vi "main_particle-filter.vi"() -> ()   [LabVIEW 2019]
uses:
  <vilib>/Analysis/Matrix/Datatypes/RealMatrix.ctl
  Ctrl/cmd_common.ctl
  <vilib>/Analysis/baseanly.llb/Real A x B.vi
  <vilib>/Analysis/Matrix/Numeric/Add/Add (Elementwise) - RM,R.vi
  <vilib>/Analysis/Matrix/NI_Matrix.lvlib
  <vilib>/ptbypt/NI_PtbyPt.lvlib
  <vilib>/Analysis/NI_AALBase.lvlib
panel:
  in  "tab":enum32{"ini val", "observation val", "Param"}(tab)=enum."observation val"
  out "Q_sim":T1=[[0.04000000000000001]]
  out "R_sim":T1=[[1.0, 0.0], [0.0, 0.2741556778080377]]
  out "x_est":T1
  out "x_true":T1
  out "h_x_est":T1
  out "h_x_dr":T1 caption="x_true"
  out "h_x_true":T1 caption="x_true"
  out "x_dr":T1
  out "R":T1=[[4.0, 0.0], [0.0, 0.4873878716587337]]
  out "Q":T1=[[0.04000000000000001]]
  in  "rf_id":cluster{"x":dbl, "y":dbl}[](array[cluster])=[{"x"=10.0, "y"=0.0}, {"x"=10.0, "y"=10.0}, {"x"=0.0, "y"=15.0}, {"x"=-5.0, "y"=20.0}]
  in  "R est err-deg":dbl=40.0 format="%#_13g"
  in  "Q est range error":dbl=0.2 format="%#_13g"
  in  "R_sim error deg":dbl=30.0 format="%#_13g"
  in  "R est in-err-distance":dbl=2.0 format="%#_13g"
  in  "Q sim range err":dbl=0.2 format="%#_13g"
  in  "R_sim range":dbl=1.0 format="%#_13g"
  out "px old":T1
  out "px new":T1
  out "p_est":T1
  out "열의 개수":i32
  in  "DT":dbl=0.1
  in  "MAX_RANGE":dbl=20.0
  in  "SIM_TIME":dbl=50.0
  in  "NTh":u32=50
  in  "NP":u32=100
  out "time":dbl
  in  "정지":bool
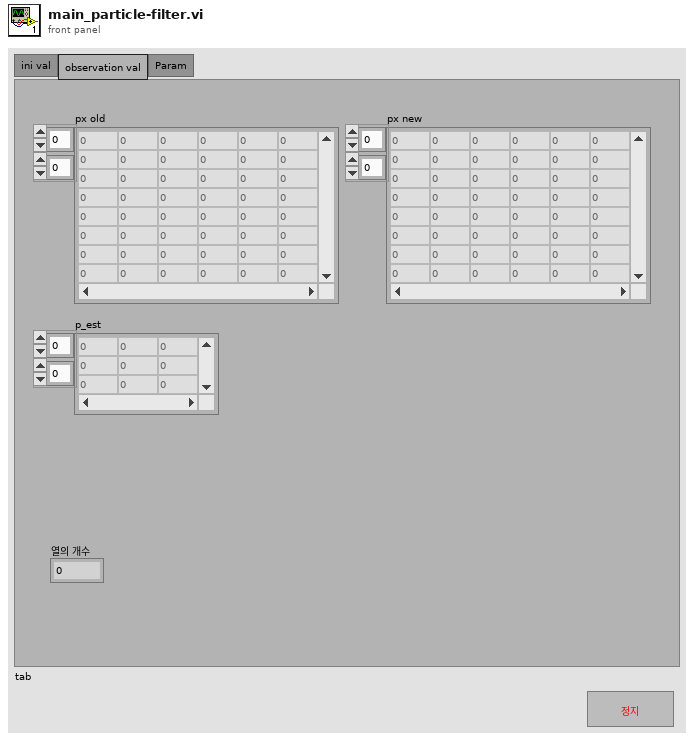
[diagram p1: front panel]
types:
  T1 = typedef "NI_Matrix.lvlib/RealMatrix.ctl" = dbl[][]
  T2 = typedef "cmd_common.ctl" = enum16{"read", "write"}
  T3 = cluster{"DT":dbl, "SIM_TIME":dbl, "MAX_RANGE":dbl, "NP":u32, "NTh":u32, T1, T1, T1, T1, "rf_id":cluster{"x":dbl, "y":dbl}[]}
  T4 = cluster{"DT":dbl, "SIM_TIME":dbl, "MAX_RANGE":dbl, "NP":u32, "NTh":u32, "Q":T1, "R":T1, "Q_sim":T1, "R_sim":T1, "rf_id":cluster{"x":dbl, "y":dbl}[]}
  T5 = cluster{"px":T1, "pw":T1, "x_dr":T1, "x_est":T1, "x_true":T1, "u":T1, "z":T1}
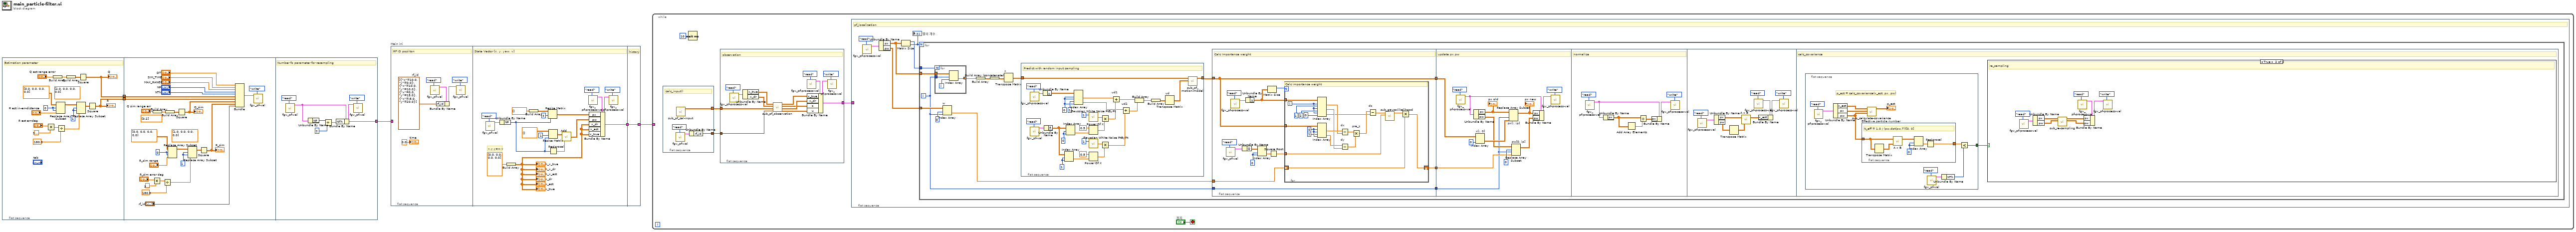
[diagram p0: block diagram]
diagram:
  n1 = flat-sequence {
    tunnel: [w7] -> w4
    tunnel: [w6] -> w3
    tunnel: w4 -> [w24]
    tunnel: w3 -> [w23]
    tunnel: [w48] -> w5
    frame #0 {
      w10 = 0 ("인덱스 (행)")
      w18 = 1 ("비활성화된 인덱스 (행)")
      (unwired) dbl[][] [[2.0, 0.0], [0.0, 0.0]] ("원소")
      # "Estimation parameter"
      n2 = Multiply(x="R est err-deg", y=3.141592653589793) -> (x*y=w19:dbl)
      n3 = Build Array("Q est range error") -> (w12:dbl[])
      n4 = Replace Array Subset(array=dbl[][] [[0.0, 0.0], [0.0, 0.0]] ("원소"), new element="R est in-err-distance", index (row)=w10, index (col)=w10) -> (w8:dbl[][])
      n5 = Divide(x=w19, y=180.0) -> (x/y=w21:dbl)
      n6 = Build Array(w12) -> (w14:T1)
      n7 = Replace Array Subset(array=w8, new element=w21, index (row)=w18, index (col)=w18) -> (w20:T1)
      n8 = Square(x=w14) -> (x^2=w7:T1)
      "Q" <- w7
      n9 = Square(x=w20) -> (x^2=w6:T1)
      "R" <- w6
    }
    frame #1 {
      w26 = 0 ("인덱스 (행)")
      w37 = 1 ("비활성화된 인덱스 (행)")
      (unwired) dbl[][] [[1.0, 0.0], [0.0, 0.0]] ("원소")
      (unwired) dbl[] [0.2] ("원소")
      n10 = Multiply(x="R_sim error deg", y=3.141592653589793) -> (x*y=w40:dbl)
      n11 = Build Array("Q sim range err") -> (w29:dbl[])
      n12 = Divide(x=w40, y=180.0) -> (x/y=w38:dbl)
      n13 = Build Array(w29) -> (w41:T1)
      n14 = Replace Array Subset(array=dbl[][] [[0.0, 0.0], [0.0, 0.0]] ("원소"), new element="R_sim range", index (row)=w26, index (col)=w26) -> (w25:dbl[][])
      n15 = Square(x=w41) -> (x^2=w33:T1)
      "Q_sim" <- w33
      n16 = Replace Array Subset(array=w25, new element=w38, index (row)=w37, index (col)=w37) -> (w39:T1)
      n17 = Square(x=w39) -> (x^2=w32:T1)
      "R_sim" <- w32
      n18 = Bundle("DT"="DT", "SIM_TIME"="SIM_TIME", "MAX_RANGE"="MAX_RANGE", "NP"="NP", "NTh"="NTh", w24, w23, w33, w32, "rf_id"="rf_id") -> (w22:T3)  [unwired: 1 in]
      n19 = call "fgv_pf-val.vi"("cmd"=cmd_common."write", "pf-val"=w22) -> ()  [unwired: 9 in, 1 out]
    }
    frame #2 {
      # "Number fo parameter for resampling"
      n20 = call "fgv_pf-val.vi"("cmd"=cmd_common."read") -> ("pf-val out"=w49:T4)  [unwired: 10 in]
      n21 = Unbundle By Name(w49) -> ("NP"=w52:u32)
      n22 = Divide(x=w52, y=u32 2) -> (x/y=w50:dbl)
      n23 = Bundle By Name(cluster=w49, "NTh"=w50) -> (w48:T4)
      n24 = call "fgv_pf-val.vi"("cmd"=cmd_common."write", "pf-val"=w48) -> ()  [unwired: 9 in, 1 out]
    }
  }
  n25 = flat-sequence "Main ini" {
    tunnel: w5 -> [_]
    tunnel: [w66] -> w1
    tunnel: [w79] -> w2
    tunnel: w1 -> [w79]
    frame #0 {
      w56 = cluster{"x":dbl, "y":dbl}[] [{"x"=10.0, "y"=0.0}, {"x"=10.0, "y"=10.0}, {"x"=0.0, "y"=15.0}, {"x"=-5.0, "y"=20.0}]  # rf_id
      # "RF ID posiiton"
      n26 = call "fgv_pf-val.vi"("cmd"=cmd_common."read") -> ("pf-val out"=w59:T4)  [unwired: 10 in]
      n27 = Bundle By Name(cluster=w59, "rf_id"=w56) -> (w60:T4)
      n28 = call "fgv_pf-val.vi"("cmd"=cmd_common."write", "pf-val"=w60) -> ()  [unwired: 9 in, 1 out]
      "time" <- 0.0 ("time")
    }
    frame #1 {
      # "x,y,yaw,v"
      # "State Vector [x, y, yaw, v]"
      n29 = call "fgv_pf-val.vi"("cmd"=cmd_common."read") -> ("pf-val out"=w77:T4)  [unwired: 10 in]
      n30 = Unbundle By Name(w77) -> ("NP"=w61:u32)
      n31 = Build Array(dbl[] [0.0, 0.0, 0.0, 0.0] ("원소")) -> (w67:T1)
      "x_est" <- w67
      "x_true" <- w67
      "x_dr" <- w67
      "h_x_true" <- w67
      "h_x_dr" <- w67
      "h_x_est" <- w67
      n32 = Build Array(dbl[] [] ("원소")) -> (w64:T1)
      n33 = Resize Matrix(1:w61, 2:4 ("행의 개수"), 4:w64) -> (0:w62:T1)
      n34 = Resize Matrix(1:w61, 2:1 ("행의 개수"), 4:T1 [] ("행렬")) -> (0:w76:T1)
      n35 = Reciprocal(x=w61) -> (1/x=w75:dbl)
      n36 = call-poly <vilib>:"Add.vi"("Real Scalar c"=w75, "Real Matrix A"=w76) -> ("A + c"=w68:T1)
      n37 = call "fgv_pf-process-val.vi"("cmd"=cmd_common."read") -> ("p-val out"=w71:T5)  [unwired: 10 in]
      n38 = Bundle By Name(cluster=w71, "px"=w62, "pw"=w68, "x_dr"=w67, "x_est"=w67, "x_true"=w67) -> (w66:T5)
      n39 = call "fgv_pf-process-val.vi"("cmd"=cmd_common."write", "p-val"=w66) -> ()  [unwired: 9 in, 1 out]
    }
    frame #2 {
      # "history"
    }
  }
  n40 = while {
    tunnel: w2 -> [_]
    stop <- "정지" stop-if-true
    n41 = flat-sequence {
      tunnel: [w251] -> w82
      tunnel: [w248] -> w81
      frame #0 {
        # "calc_input()"
        n42 = call "fgv_pf-val.vi"("cmd"=cmd_common."read") -> ("pf-val out"=w249:T4)  [unwired: 10 in]
        n43 = call "sub_pf_cal-input.vi"() -> ("Real Matrix"=w251:T1)  [unwired: 11 in]
        n44 = Unbundle By Name(w249) -> ("rf_id"=w248:cluster{"x":dbl, "y":dbl}[])
      }
    }
    n45 = Wait (ms)(milliseconds to wait=u32 10 ("대기 시간 (ms)")) -> ()  [unwired: 1 out]
    n46 = flat-sequence {
      tunnel: w82 -> [w98]
      tunnel: w81 -> [w97]
      tunnel: [w85] -> w80
      frame #0 {
        # "observation"
        n47 = call "fgv_pf-process-val.vi"("cmd"=cmd_common."read") -> ("p-val out"=w90:T5)  [unwired: 10 in]
        n48 = Unbundle By Name(w90) -> ("x_true"=w89:T1, "x_dr"=w88:T1)
        n49 = call "sub_pf_observation.vi"("rf_id"=w97, "u"=w98, "xd"=w88, "x_true"=w89) -> ("ud"=w87:T1, "xd out"=w92:T1, "z"=w86:T1, "x_true out"=w93:T1)  [unwired: 4 in]
        n50 = call "fgv_pf-process-val.vi"("cmd"=cmd_common."read") -> ("p-val out"=w94:T5)  [unwired: 10 in]
        n51 = Bundle By Name(cluster=w94, "x_true"=w93, "x_dr"=w92, "z"=w86, "u"=w87) -> (w85:T5)
        n52 = call "fgv_pf-process-val.vi"("cmd"=cmd_common."write", "p-val"=w85) -> ()  [unwired: 9 in, 1 out]
      }
    }
    n53 = flat-sequence {
      tunnel: w80 -> [_]
      frame #0 {
        # "pf_localization"
        n54 = call "fgv_pf-process-val.vi"("cmd"=cmd_common."read") -> ("p-val out"=w102:T5)  [unwired: 10 in]
        n55 = Unbundle By Name(w102) -> ("px"=w101:T1, "pw"=w99:T1)
        n56 = Matrix Size(0:w101) -> (1:w100:i32, 2:w104:i32)
        "열의 개수" <- w104
        n57 = for {
          N: w104 -> [_]
          tunnel: w101 -> [w118]
          tunnel: w100 -> [w117]
          tunnel: w99 -> [w116]
          i -> [w108]
          n58 = for {
            N: w117 -> [_]
            tunnel: w118 -> [w247]
            tunnel: w108 -> [w245]
            tunnel: [w244] -> w112 mode=indexing
            i -> [w246]
            n59 = Index Array(array=w247, index (row)=w245, index (col)=w246) -> (element=w244:dbl)
          }
          n60 = Index Array "w"(array=w116, index (row)=0 ("인덱스 (행)"), index (col)=w108) -> (element=w109:dbl)
          n61 = Build Array(w112) -> (w114:dbl[][])
          n62 = Build Array (concatenate)(w114) -> (w113:T1)
          n63 = Transpose Matrix "x"(1:w113) -> (0:w111:T1)
          n64 = flat-sequence {
            tunnel: w111 -> [w144]
            tunnel: [w119] -> w110
            frame #0 {
              w129 = 1 ("인덱스 (행)")
              w140 = 0 ("인덱스 (행)")
              w145 = 0 ("인덱스 (행)")
              # "Predict with random input sampling"
              n65 = call "fgv_pf-process-val.vi"("cmd"=cmd_common."read") -> ("p-val out"=w148:T5)  [unwired: 10 in]
              n66 = call "fgv_pf-val.vi"("cmd"=cmd_common."read") -> ("pf-val out"=w141:T4)  [unwired: 10 in]
              n67 = Unbundle By Name(w148) -> ("u"=w147:T1)
              n68 = Unbundle By Name(w141) -> ("R"=w120:T1)
              n69 = Index Array(array=w120, index (row)=w129, index (col)=w129) -> (element=w130:dbl)
              n70 = Index Array(array=w120, index (row)=w140, index (col)=w140) -> (element=w139:dbl)
              n71 = Index Array(array=w147, index (row) #1=w145, index (col) #1=w145, index (row) #2=1 ("인덱스 (행)"), index (col) #2=w145) -> (element #1=w134:dbl, element #2=w127:dbl)
              n72 = call <vilib>:"Gaussian White Noise PtByPt.vi"("standard deviation"=1 ("samples")) -> ("Gaussian white noise"=w136:dbl)  [unwired: 2 in]
              n73 = Power Of X(1:w139, 2:0.5 ("y")) -> (0:w137:dbl)
              n74 = call <vilib>:"Gaussian White Noise PtByPt.vi"("standard deviation"=1 ("samples")) -> ("Gaussian white noise"=w133:dbl)  [unwired: 2 in]
              n75 = Power Of X(1:w130, 2:0.5 ("y")) -> (0:w132:dbl)
              n76 = Multiply(x=w136, y=w137) -> (x*y=w135:dbl)
              n77 = Multiply(x=w133, y=w132) -> (x*y=w126:dbl)
              n78 = Add "ud1"(x=w134, y=w135) -> (x+y=w122:dbl)
              n79 = Add "ud2"(x=w127, y=w126) -> (x+y=w123:dbl)
              n80 = Build Array(w122, w123) -> (w124:dbl[])
              n81 = Build Array(w124) -> (w125:T1)
              n82 = Transpose Matrix "ud"(1:w125) -> (0:w121:T1)
              n83 = call "sub_pf_motion-model.vi"("u"=w121, "x_true"=w144) -> ("x_true out"=w119:T1)  [unwired: 9 in]
            }
          }
          n84 = flat-sequence {
            tunnel: w110 -> [w151]
            tunnel: w109 -> [w153]
            tunnel: w108 -> [w152]
            tunnel: [w152] -> w107
            tunnel: [w151] -> w106
            tunnel: [w150] -> w105
            tunnel: w107 -> [w186]
            tunnel: w106 -> [w194]
            tunnel: w105 -> [w187]
            frame #0 {
              w156 = 0 ("인덱스 (행)")
              # "Calc Importance weight"
              n85 = call "fgv_pf-val.vi"("cmd"=cmd_common."read") -> ("pf-val out"=w158:T4)  [unwired: 10 in]
              n86 = call "fgv_pf-process-val.vi"("cmd"=cmd_common."read") -> ("p-val out"=w162:T5)  [unwired: 10 in]
              n87 = Unbundle By Name(w158) -> ("Q"=w157:T1)
              n88 = Unbundle By Name(w162) -> ("z"=w160:T1)
              n89 = Index Array(array=w157, index (row)=w156, index (col)=w156) -> (element=w155:dbl)
              n90 = Matrix Size(0:w160) -> (1:w161:i32)  [unwired: 1 out]
              n91 = Square Root(x=w155) -> (sqrt(x)=w154:dbl)
              n92 = for {
                N: w161 -> [_]
                tunnel: w151 -> [w184]
                tunnel: w160 -> [w181]
                tunnel: w154 -> [w168]
                shift-right: [w164] -> w150
                shift-left: w153 -> [w165]
                i -> [w167]
                w183 = 0 ("인덱스 (행)")
                # "Calc importance weight"
                n93 = Index Array(array=w181, index (row) #1=w167, index (col) #1=1 ("인덱스 (열)"), index (row) #2=w167, index (col) #2=2 ("인덱스 (열)"), index (row) #3=w167, index (col) #3=0 ("인덱스 (열)")) -> (element #1=w177:dbl, element #2=w175:dbl, element #3=w170:dbl)
                n94 = Index Array(array=w184, index (row) #1=w183, index (col) #1=w183, index (row) #2=1 ("인덱스 (행)"), index (col) #2=w183) -> (element #1=w178:dbl, element #2=w176:dbl)
                n95 = Subtract "dx"(x=w178, y=w177) -> (x-y=w173:dbl)
                n96 = Subtract "dy"(x=w176, y=w175) -> (x-y=w174:dbl)
                n97 = Multiply "pre_z"(x=w173, y=w174) -> (x*y=w171:dbl)
                n98 = Subtract "dz"(x=w171, y=w170) -> (x-y=w169:dbl)
                n99 = call "sub_gauss-likelihood.vi"("sigma"=w168, "x"=w169) -> ("p"=w166:dbl)  [unwired: 9 in]
                n100 = Multiply ("Multiply.vi")(x=w166, y=w165) -> (x*y=w164:dbl)
              }
            }
            frame #1 {
              # "update px,pw"
              n101 = call "fgv_pf-process-val.vi"("cmd"=cmd_common."read") -> ("p-val out"=w195:T5)  [unwired: 10 in]
              n102 = Unbundle By Name(w195) -> ("px"=w192:T1, "pw"=w189:T1)
              "px old" <- w192
              n103 = Index Array "x[:, 0]"(array=w194, index (col)=0) -> (element=w191:T1)  [unwired: 1 in]
              n104 = Replace Array Subset "px[:, ip]"(array=w192, new element=w191, index (col)=w186) -> (w190:T1)  [unwired: 1 in]
              "px new" <- w190
              n105 = Replace Array Subset "pw[0, ip]"(array=w189, new element=w187, index (row)=0 ("index (col)"), index (col)=w186) -> (w185:T1)
              n106 = Bundle By Name(cluster=w195, "px"=w190, "pw"=w185) -> (w198:T5)
              n107 = call "fgv_pf-process-val.vi"("cmd"=cmd_common."write", "p-val"=w198) -> ()  [unwired: 9 in, 1 out]
            }
            frame #2 {
              # "normalize"
              n108 = call "fgv_pf-process-val.vi"("cmd"=cmd_common."read") -> ("p-val out"=w202:T5)  [unwired: 10 in]
              n109 = Unbundle By Name(w202) -> ("px"=w200:T1)
              n110 = Add Array Elements(numeric array=w200) -> (sum=w199:dbl)
              n111 = Divide(x=w200, y=w199) -> (x/y=w201:T1)
              n112 = Bundle By Name(cluster=w202, "px"=w201) -> (w205:T5)
              n113 = call "fgv_pf-process-val.vi"("cmd"=cmd_common."write", "p-val"=w205) -> ()  [unwired: 9 in, 1 out]
            }
            frame #3 {
              n114 = call "fgv_pf-process-val.vi"("cmd"=cmd_common."read") -> ("p-val out"=w215:T5)  [unwired: 10 in]
              n115 = Unbundle By Name(w215) -> ("px"=w213:T1, "pw"=w212:T1)
              n116 = Transpose Matrix(1:w212) -> (0:w211:T1)
              n117 = call-poly <vilib>:"A x B.vi"("B"=w211, "A"=w213) -> ("A x B"=w206:T1)  [unwired: 1 out]
              n118 = call "fgv_pf-process-val.vi"("cmd"=cmd_common."read") -> ("p-val out"=w209:T5)  [unwired: 10 in]
              n119 = Bundle By Name(cluster=w209, "x_est"=w206) -> (w210:T5)
              n120 = call "fgv_pf-process-val.vi"("cmd"=cmd_common."write", "p-val"=w210) -> ()  [unwired: 9 in, 1 out]
            }
            frame #4 {
              # "calc_covariance"
              n121 = flat-sequence {
                tunnel: [w217] -> w216
                frame #0 {
                  # "p_est = calc_covariance(x_est, px, pw)"
                  n122 = call "fgv_pf-process-val.vi"("cmd"=cmd_common."read") -> ("p-val out"=w226:T5)  [unwired: 10 in]
                  n123 = Unbundle By Name(w226) -> ("x_est"=w224:T1, "px"=w225:T1, "pw"=w222:T1)
                  n124 = flat-sequence "Effective particle number" {
                    tunnel: w222 -> [w233]
                    tunnel: [w228] -> w220
                    frame #0 {
                      w230 = 0 ("index (row)")
                      # "N_eff = 1.0 / (pw.dot(pw.T))[0, 0]"
                      n125 = Transpose Matrix(1:w233) -> (0:w232:T1)
                      n126 = call-poly <vilib>:"A x B.vi"("B"=w232, "A"=w233) -> ("A x B"=w231:T1)  [unwired: 1 out]
                      n127 = Index Array(array=w231, index (row)=w230, index (col)=w230) -> (element=w229:dbl)
                      n128 = Reciprocal(x=w229) -> (1/x=w228:dbl)
                    }
                  }
                  n129 = call "sub_calculate-covariance.vi"("pw"=w222, "px"=w225, "x_est"=w224) -> ("cov out"=→"p_est":T1)  [unwired: 8 in]
                  n130 = call "fgv_pf-val.vi"("cmd"=cmd_common."read") -> ("pf-val out"=w219:T4)  [unwired: 10 in]
                  n131 = Unbundle By Name(w219) -> ("NTh"=w218:u32)
                  n132 = Less?(x=w220, y=w218) -> (x < y?=w217:bool)
                }
              }
              n133 = case shown="True" w216 {
                frame False {
                }
                frame True {
                  # "re_sampling"
                  n134 = call "fgv_pf-process-val.vi"("cmd"=cmd_common."read") -> ("p-val out"=w243:T5)  [unwired: 10 in]
                  n135 = Unbundle By Name(w243) -> ("px"=w240:T1, "pw"=w241:T1)
                  n136 = call "sub_re-sampling.vi"("pw"=w241, "px"=w240) -> ("A + c"=w234:T1, "Real Matrix"=w235:T1)  [unwired: 8 in]
                  n137 = call "fgv_pf-process-val.vi"("cmd"=cmd_common."read") -> ("p-val out"=w238:T5)  [unwired: 10 in]
                  n138 = Bundle By Name(cluster=w238, "px"=w235, "pw"=w234) -> (w239:T5)
                  n139 = call "fgv_pf-process-val.vi"("cmd"=cmd_common."write", "p-val"=w239) -> ()  [unwired: 9 in, 1 out]
                }
              }
            }
          }
        }
      }
    }
  }
